vi "getSettingFilePaths.vi"(11 "Setting in":refnum<class "Setting.lvclass">) -> (2 "SettingFilePaths":path[](array[path]), 3 "Setting out":refnum<class "Setting.lvclass">)   [LabVIEW 2016, in "Setting.lvclass"]
uses:
  Setting.lvclass
  Setting.lvclass/Setting.ctl
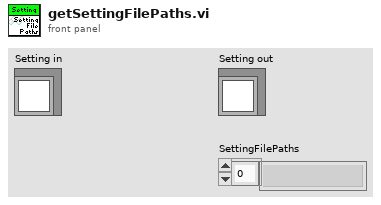
[diagram p1: front panel]
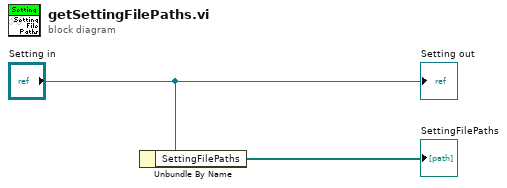
[diagram p0: block diagram]
diagram:
  n1 = Unbundle By Name("Setting in") -> ("SettingFilePaths"=→"SettingFilePaths":path[])
  "Setting out" <- "Setting in"
